vi "ExReadFileHeaderTimeStamp.vi"(5 "error in (no error)":errorcluster) -> (4 "error out":errorcluster)   [LabVIEW 2010]
panel:
  out "Time per Frame (tics)":dbl
  out "UTC End":string
  out "UTC Start":string
  out "Date End":string
  out "Date Start":string
  out "Tics Elapsed":u64
  out "Tics End":u64
  out "Tics Start":u64
  in  "Full File Name":path
  in  "FileType":u32=67633152
  # "ExReadFileHeaderTimeStamp.vi\nThis VI will use read time stamp information stored in the file header and display it."
  # "File Types:\nSPE = 67371008\nTIF  = 67174400\nPMI = 67436544\nR3B = 67633152"
  # "Browse match pattern is set to *.r3b.  Modify this if different file type is needed."
  # "Start Time (tics)"
  # "End Time (tics)"
  # "Elapsed Time (tics)"
  # "Time Per Frame (tics)"
  # "Local"
  # "UTC"
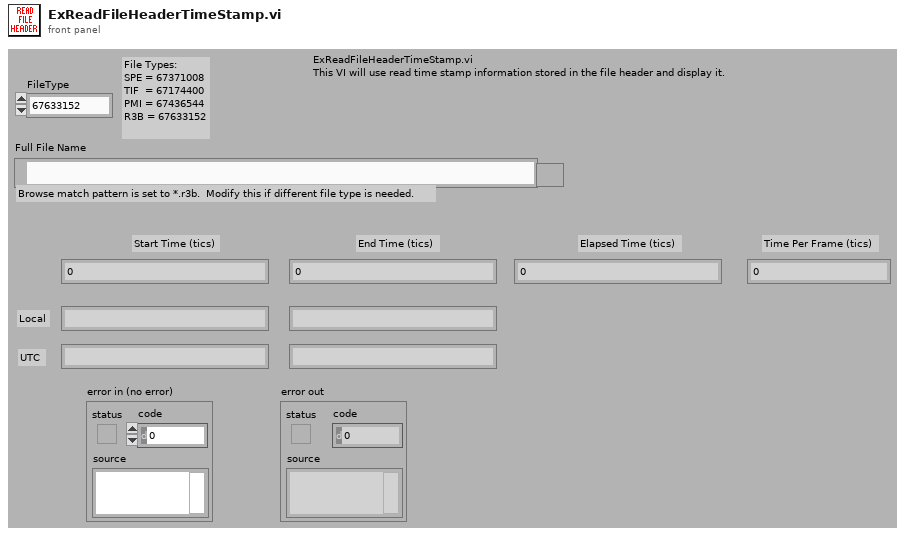
[diagram p1: front panel]
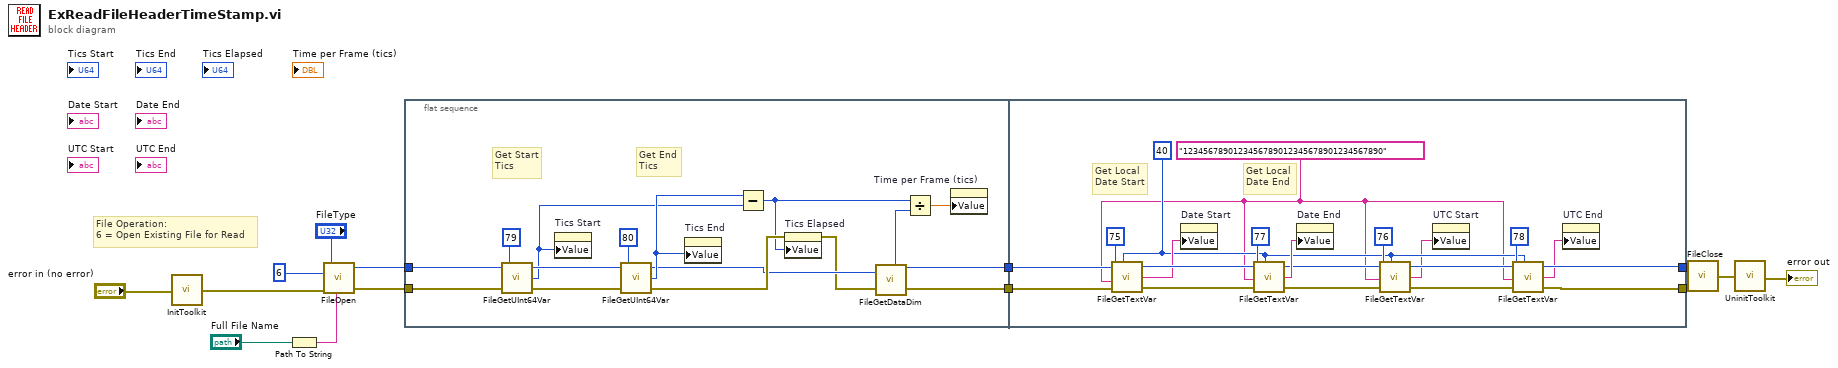
[diagram p0: block diagram]
diagram:
  # "File Operation:\n6 = Open Existing File for Read"
  n1 = call <userlib>:"InitToolkit.vi"("error in"="error in (no error)") -> ("error out"=w13:errorcluster)
  n2 = Path To String(path="Full File Name") -> (string=w12:string)
  n3 = call <userlib>:"FileOpen.vi"("error in"=w13, "File Operations"=u32 6 ("File Operation"), "FileName"=w12, "File Type"="FileType") -> ("error out"=w1:errorcluster, "File Handle"=w2:u32)
  n4 = flat-sequence {
    tunnel: w2 -> [w30]
    tunnel: w1 -> [w29]
    tunnel: [w20] -> w6
    tunnel: [w18] -> w5
    tunnel: [w47] -> _
    tunnel: [w48] -> w4
    tunnel: w6 -> [w49]
    tunnel: w5 -> [w50]
    tunnel: [w47] -> w3
    frame #0 {
      # "Get End\nTics"
      # "Get Start\nTics"
      n5 = call <userlib>:"FileGetUInt64Var.vi"("error in"=w29, "Parameter ID"=79, "File Handle"=w30) -> ("error out"=w25:errorcluster, "Value"=w22:u64, "File Handle"=w26:u32)
      n6 = property on="Tics Start" class="DigNum (strict)"("Value"=w22) -> ()  [unwired: 2 in, 2 out]
      n7 = call <userlib>:"FileGetUInt64Var.vi"("error in"=w25, "Parameter ID"=80, "File Handle"=w26) -> ("error out"=w24:errorcluster, "Value"=w23:u64, "File Handle"=w21:u32)
      n8 = property on="Tics End" class="DigNum (strict)"("Value"=w23) -> ()  [unwired: 2 in, 2 out]
      n9 = Subtract(x=w23, y=w22) -> (x-y=w17:u64)
      n10 = property on="Tics Elapsed" class="DigNum (strict)"(error in=w24, "Value"=w17) -> (error out=w19:errorcluster)  [unwired: 1 in, 1 out]
      n11 = call <userlib>:"FileGetDataDim.vi"("File Handle"=w21, "error in"=w19) -> ("Number of Frames"=w16:u32, "File Handle"=w20:u32, "error out"=w18:errorcluster)  [unwired: 3 out]
      n12 = Divide(x=w17, y=w16) -> (x/y=w15:dbl)
      n13 = property on="Time per Frame (tics)" class="DigNum (strict)"("Value"=w15) -> ()  [unwired: 2 in, 2 out]
    }
    frame #1 {
      w34 = 40
      w33 = "1234567890123456789012345678901234567890"
      # "Get Local\nDate End"
      # "Get Local\nDate Start"
      n14 = call <userlib>:"FileGetTextVar.vi"("File Handle"=w49, "Parameter ID"=75, "User Text Buffer"=w33, "error in"=w50, "Text Buffer Size"=w34) -> ("File Handle"=w44:u32, "Text Value Returned"=w42:string, "error out"=w43:errorcluster)
      n15 = property on="Date Start" class="Str"("Value"=w42) -> ()  [unwired: 2 in, 2 out]
      n16 = call <userlib>:"FileGetTextVar.vi"("File Handle"=w44, "Parameter ID"=77, "User Text Buffer"=w33, "error in"=w43, "Text Buffer Size"=w34) -> ("File Handle"=w38:u32, "Text Value Returned"=w41:string, "error out"=w36:errorcluster)
      n17 = property on="Date End" class="Str"("Value"=w41) -> ()  [unwired: 2 in, 2 out]
      n18 = call <userlib>:"FileGetTextVar.vi"("File Handle"=w38, "Parameter ID"=76, "User Text Buffer"=w33, "error in"=w36, "Text Buffer Size"=w34) -> ("File Handle"=w37:u32, "Text Value Returned"=w32:string, "error out"=w35:errorcluster)
      n19 = property on="UTC Start" class="Str"("Value"=w32) -> ()  [unwired: 2 in, 2 out]
      n20 = call <userlib>:"FileGetTextVar.vi"("File Handle"=w37, "Parameter ID"=78, "User Text Buffer"=w33, "error in"=w35, "Text Buffer Size"=w34) -> ("File Handle"=w48:u32, "Text Value Returned"=w31:string, "error out"=w47:errorcluster)
      n21 = property on="UTC End" class="Str"("Value"=w31) -> ()  [unwired: 2 in, 2 out]
    }
  }
  n22 = call <userlib>:"FileClose.vi"("error in"=w3, "File Handle"=w4) -> ("error out"=w7:errorcluster)
  n23 = call <userlib>:"UninitToolkit.vi"("error in"=w7) -> ("error out"=→"error out":errorcluster)
